vi "Position_Based_L4_Motion_deg.vi"(8 "assign z":dbl, 9 "EyeCenter x val":dbl, 10 "current z":dbl, 11 "current x":dbl) -> (3 "L4 motion [deg]":dbl)   [LabVIEW 2010]
doc: "This VI calculates the L4 motion based on the current (x,~,z) position.\nIt is designed so that the aspiration hole is always facing towards a virtual axis (EyeCenter x val,~,assign z)."
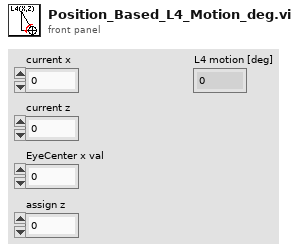
[diagram p1: front panel]
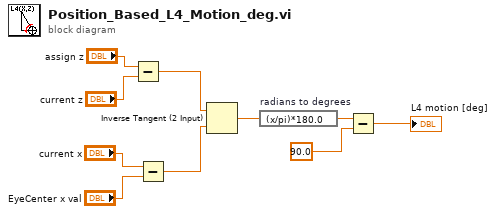
[diagram p0: block diagram]
diagram:
  n1 = Subtract(x="assign z", y="current z") -> (x-y=w6:dbl)
  n2 = Subtract(x="current x", y="EyeCenter x val") -> (x-y=w5:dbl)
  n3 = Inverse Tangent (2 Input)(1:w5, 2:w6) -> (0:w4:dbl)
  n4 = expression code="(x/pi)*180.0" "radians to degrees"(w4) -> (w3:dbl)
  n5 = Subtract(x=w3, y=90.0) -> (x-y=→"L4 motion [deg]":dbl)
